vi "View.vi"(8 "error in (no error)":errorcluster, 11 "Worker In":refnum<class "Worker.lvclass">) -> (0 "error out":errorcluster, 3 "Worker Out":refnum<class "Worker.lvclass">)   [LabVIEW 2020, in "Worker.lvclass"]
doc: "This VI implements the main UI of the process. A reference to this VI should be set using the Set View VI Reference.vi method when the VI is started."
uses:
  Worker.lvclass
  C:/Program Files (x86)/National Instruments/LabVIEW 2020/vi.lib/Asteme/Triarc Framework/Process/Process.lvclass
  C:/Program Files (x86)/National Instruments/LabVIEW 2020/vi.lib/Asteme/Triarc Framework/View/View.lvclass
  <vilib>/Asteme/Triarc Framework/View/View.lvclass/View.ctl
  <vilib>/Asteme/Triarc Framework/Process/Process.lvclass/Process.ctl
  <vilib>/Asteme/Triarc Framework/Process/Protected/Messaging/Enqueue Message.vi
  <vilib>/AdvancedString/1D String Array to Delimited String.vi
  <vilib>/Asteme/Triarc Framework/Process/Public/Lifecycle/Get Lifecycle State.vi
  <vilib>/Utility/error.llb/Clear Errors.vi
  <vilib>/Utility/error.llb/Error Cluster From Error Code.vi
  <vilib>/Asteme/Triarc Framework/Process/Process.lvclass
  <vilib>/Asteme/Triarc Framework/View/View.lvclass
panel:
  out "Name":string
  out "Worker Type":string="Barista"
  out "Orders Filled This Shift":u32
  out "Status":string
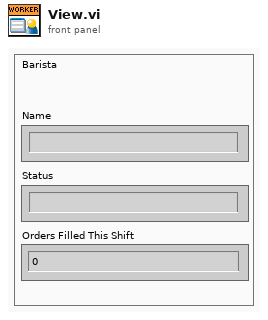
[diagram p1: front panel]
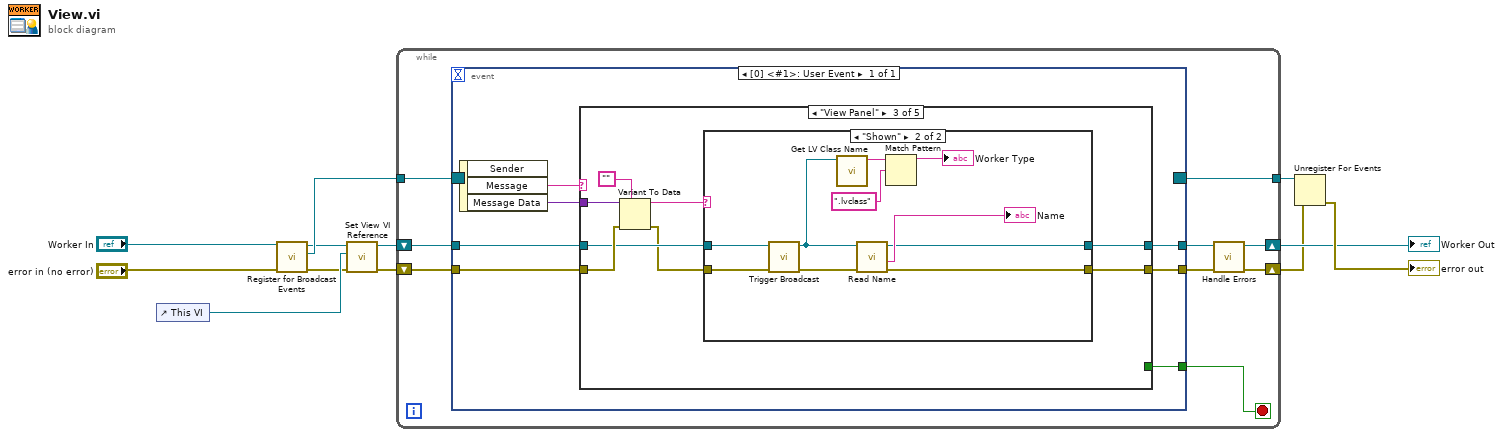
[diagram p0: block diagram]
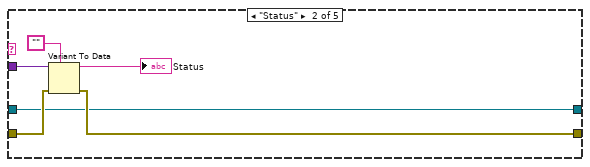
[diagram p3: hidden frame]
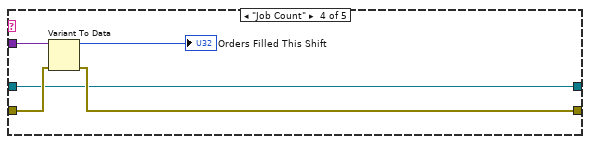
[diagram p5: hidden frame]
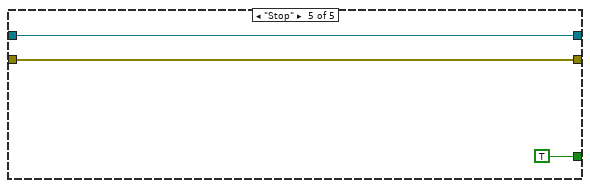
[diagram p6: hidden frame]
diagram:
  n1 = control-ref of="This VI"() -> (w10:refnum<vi>)
  n2 = call <vilib>:"Register for Broadcast Events.vi"("error in (no error)"="error in (no error)", "Process In"="Worker In") -> ("error out"=w8:errorcluster, "Event Registration Refnum Out"=w9:refnum<event-registration>, "Process Out"=w7:refnum<class "Worker.lvclass">)  [unwired: 7 in]
  n3 = call <vilib>:"Set View VI Reference.vi"("error in (no error)"=w8, "View VI Reference"=w10, "UI View in"=w7) -> ("error out"=w6:errorcluster, "UI View out"=w5:refnum<class "Worker.lvclass">)  [unwired: 7 in]
  n4 = while {
    shift-right: [w15] -> w11
    shift-left: w5 -> [w21]
    shift-right: [w13] -> w4
    shift-left: w6 -> [w19]
    tunnel: w9 -> [w18]
    tunnel: [w17] -> w3
    stop <- w16 stop-if-true
    n5 = event shown="[0] <#1>: User Event" {
      selector: w18 -> [_]
      dyn-events: [_] -> w17
      timeout: _ -> [_]
      tunnel: w21 -> [w28]
      tunnel: [w27] -> w20
      tunnel: w19 -> [w25]
      tunnel: [w26] -> w14
      tunnel: [w23] -> w16
      event User Event {
        n6 = event-data() -> ("Message"=w24:string, "Message Data"=w22:variant)  [unwired: 1 in, 1 out]
        n7 = case shown="\"View Panel\"" w24 {
          tunnel: w28 -> [w30 w31 w40 w58 w64]
          tunnel: [w30 w31 w39 w58 w64] -> w27
          tunnel: [w29 w32 w37 w59 w63] -> w26
          tunnel: w25 -> [w29 w35 w43 w60 w63]
          tunnel: [_ _ _ _ TRUE] -> w23
          tunnel: w22 -> [_ w36 w44 w61 _]
          frame Default {
          }
          frame "Status" {
            n8 = Variant To Data(error in=w35, type="", Variant=w36) -> (data=→"Status":string, error out=w32:errorcluster)
          }
          frame "View Panel" {
            n9 = Variant To Data(error in=w43, type="", Variant=w44) -> (data=w41:string, error out=w38:errorcluster)
            n10 = case shown="\"Shown\"" w41 {
              tunnel: w40 -> [w46 w48]
              tunnel: [w46 w52] -> w39
              tunnel: w38 -> [w45 w51]
              tunnel: [w45 w50] -> w37
              frame Default {
              }
              frame "Shown" {
                n11 = call <vilib>:"Trigger Broadcast.vi"("error in (no error)"=w51, "Process in"=w48) -> ("error out"=w49:errorcluster, "Process out"=w47:refnum<class "Worker.lvclass">)  [unwired: 8 in]
                n12 = call <vilib>:"Get LV Class Name.vi"("object"=w47) -> ("class name"=w54:string)  [unwired: 9 in, 1 out]
                n13 = call-dynamic "Read Name.vi"("error in (no error)"=w49, "Process In"=w47) -> ("error out"=w50:errorcluster, "Name"=→"Name":string, "Process Out"=w52:refnum<class "Worker.lvclass">)  [unwired: 6 in, 1 out]
                n14 = Match Pattern(string=w54, regular expression=".lvclass") -> (before substring=→"Worker Type":string)  [unwired: 1 in, 3 out]
              }
            }
          }
          frame "Job Count" {
            n15 = Variant To Data(error in=w60, Variant=w61) -> (data=→"Orders Filled This Shift":u32, error out=w59:errorcluster)  [unwired: 1 in]
          }
          frame "Stop" {
          }
        }
      }
    }
    n16 = call-dynamic "Handle Errors.vi"("error in (no error)"=w14, "Process In"=w20) -> ("error out"=w13:errorcluster, "Process Out"=w15:refnum<class "Worker.lvclass">)  [unwired: 8 in]
  }
  "Worker Out" <- w11
  n17 = Unregister For Events(event registration refnum=w3, error in=w4) -> (error out=→"error out":errorcluster)
